vi "Next Open.vi"(11 "Map In":T1) -> (1 "Empty?":bool, 2 "Position":cluster{"Row":i32, "Col":i32}, 3 "Map":T1)   [LabVIEW 2022 SP3, in "AoC22.lvlib"]
uses:
  AoC22.lvlib
  Map.ctl
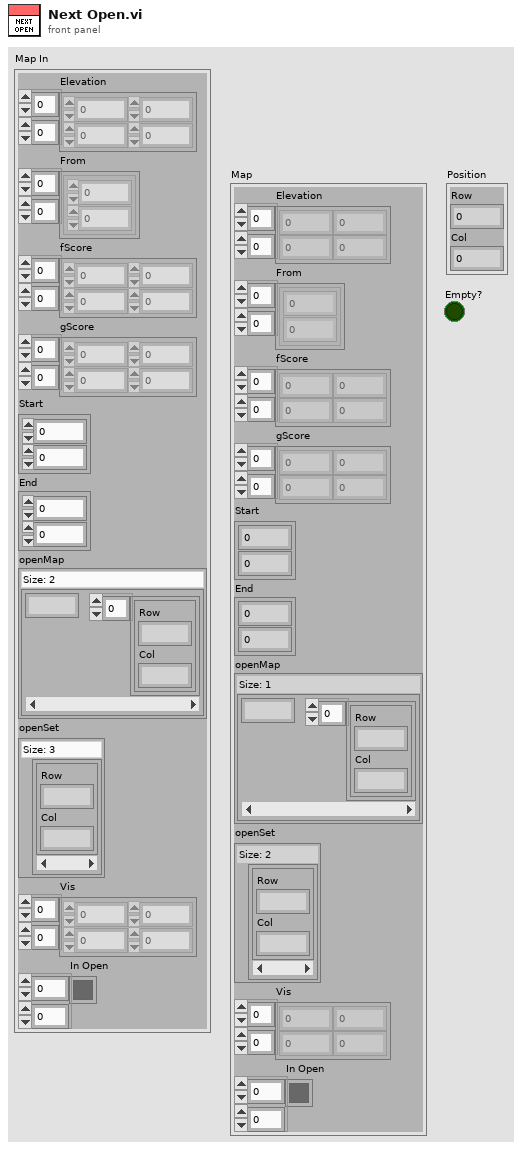
[diagram p1: front panel]
types:
  T1 = typedef "AoC22.lvlib/Map.ctl" = cluster{"Elevation":u8[][], "From":cluster{"Row":i32, "Col":i32}[][], "fScore":i32[][], "gScore":i32[][], "Start":cluster{"Row":i32, "Col":i32}, "End":cluster{"Row":i32, "Col":i32}, "openMap":map{i32, cluster{"Row":i32, "Col":i32}[]}, "openSet":set{cluster{"Row":i32, "Col":i32}}, "Vis":u8[][], "In Open":bool[][]}
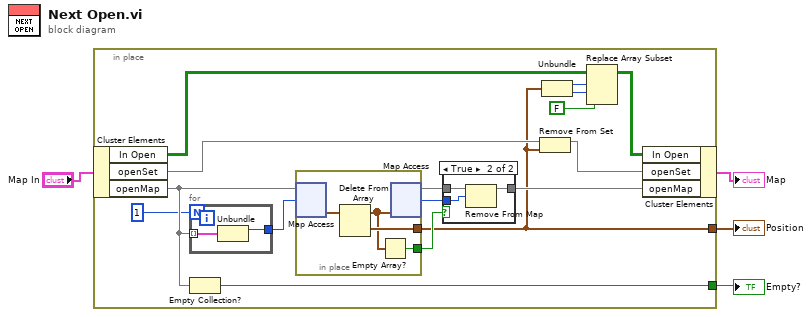
[diagram p0: block diagram]
diagram:
  n1 = in-place {
    in-place-border: [w20] -> w4
    in-place-border: [w10] -> w2
    n2 = in-place-cluster #1("Map In") -> ("In Open"=w9:bool[][], "openSet"=w11:set{cluster{"Row":i32, "Col":i32}}, "openMap"=w19:map{i32, cluster{"Row":i32, "Col":i32}[]})
    n3 = for {
      N: 1 -> [_]
      tunnel: w19 -> [w30] mode=indexing
      tunnel: [w29] -> w17
      n4 = Unbundle(w30) -> ("fScore"=w29:i32)  [unwired: 1 out]
    }
    n5 = Empty Collection?(1:w19) -> (0:w20:bool)
    n6 = in-place {
      in-place-border: [w28] -> w10
      in-place-border: [w25] -> w13
      n7 = in-place-map #2(w19, w17) -> (w27:cluster{"Row":i32, "Col":i32}[])  [unwired: 1 in, 1 out]
      n8 = Delete From Array(array=w27) -> (deleted portion=w28:cluster{"Row":i32, "Col":i32}, array with subset deleted=w26:cluster{"Row":i32, "Col":i32}[])  [unwired: 2 in]
      n9 = Empty Array?(array=w26) -> (empty?=w25:bool)
      n10 = in-place-map #2(w26) -> (w16:map{i32, cluster{"Row":i32, "Col":i32}[]}, w14:i32)  [unwired: 1 in, 1 out]
    }
    n11 = case shown="True" w13 {
      tunnel: w16 -> [w21 w24]
      tunnel: [w21 w23] -> w15
      tunnel: w14 -> [_ w22]
      frame False {
      }
      frame True {
        n12 = Remove From Map(10:w22, 11:w24) -> (3:w23:map{i32, cluster{"Row":i32, "Col":i32}[]})  [unwired: 2 out]
      }
    }
    n13 = Remove From Set(10:w10, 11:w11) -> (3:w12:set{cluster{"Row":i32, "Col":i32}})  [unwired: 1 out]
    n14 = Unbundle(w10) -> ("Row"=w6:i32, "Col"=w5:i32)
    n15 = Replace Array Subset(array=w9, new element=FALSE ("new element/subarray"), index (row)=w6, index (col)=w5) -> (w7:bool[][])
    n16 = in-place-cluster #1("In Open"=w7, "openSet"=w12, "openMap"=w15) -> (→"Map":T1)
  }
  "Empty?" <- w4
  "Position" <- w2
